vi "Labspec GetActiveData.vi"(8 "error in":errorcluster, 10 "Data Type":T1(ring), 11 "Automation Refnum In":refnum<k7>) -> (0 "error out":errorcluster, 1 "No Active Data?":bool, 2 "Data ID":i32, 3 "Automation Refnum Out":refnum<k7>)   [LabVIEW 2014]
panel:
  # "LICENSED MATERIALS – PROPERTY OF IBM\nCopyright IBM Corp. 2016,\nALL RIGHTS RESERVED"
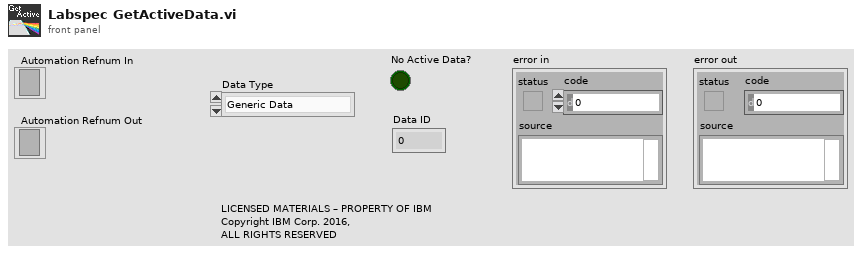
[diagram p1: front panel]
types:
  T1 = enum16{"Generic Data", "Spectrum", "Spectral Profile Image", "Map", "Video", "First Data", "Next Data"}
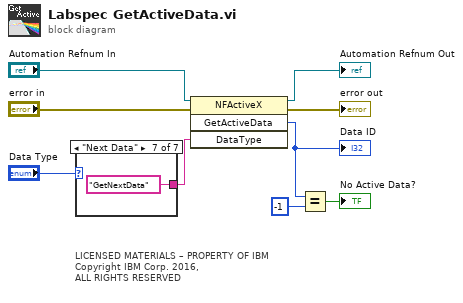
[diagram p0: block diagram]
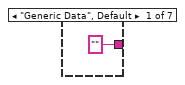
[diagram p2: hidden frame]
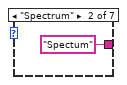
[diagram p3: hidden frame]
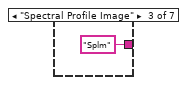
[diagram p4: hidden frame]
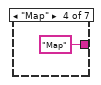
[diagram p5: hidden frame]
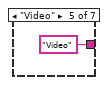
[diagram p6: hidden frame]
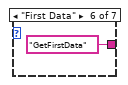
[diagram p7: hidden frame]
diagram:
  # "LICENSED MATERIALS – PROPERTY OF IBM\nCopyright IBM Corp. 2016,\nALL RIGHTS RESERVED"
  n1 = case shown="\"Next Data\"" "Data Type" {
    tunnel: ["" ("DataType") "Spectum" ("DataType") "Splm" ("DataType") "Map" ("DataType") "Video" ("DataType") "GetFirstData" ("DataType") "GetNextData" ("DataType")] -> w1
    frame "Generic Data", Default {
    }
    frame "Spectrum" {
    }
    frame "Spectral Profile Image" {
    }
    frame "Map" {
    }
    frame "Video" {
    }
    frame "First Data" {
    }
    frame "Next Data" {
    }
  }
  n2 = invoke class="NFActiveX" method="GetActiveData"(reference="Automation Refnum In", error in="error in", "DataType"=w1) -> (reference out=→"Automation Refnum Out":refnum<k7>, error out=→"error out":errorcluster, "GetActiveData"=w4:i32)  [unwired: 1 in, 1 out]
  "Data ID" <- w4
  n3 = Equal?(x=w4, y=-1) -> (x = y?=→"No Active Data?":bool)
